vi "Open.vi"(5 "LogEnabled":bool, 7 "LogPath":path, 8 "error in (no error)":errorcluster, 9 "Instance":string, 10 "BaudRate":u32=125000, 11 "GenericCanAdapterClass in":refnum<class "GenericCanAdapterClass.lvclass">) -> (0 "error out":errorcluster, 3 "GenericCanAdapterClass out":refnum<class "GenericCanAdapterClass.lvclass">)   [LabVIEW 2011, in "GenericCanAdapterClass.lvclass"]
uses:
  GenericCanAdapterClass.lvclass
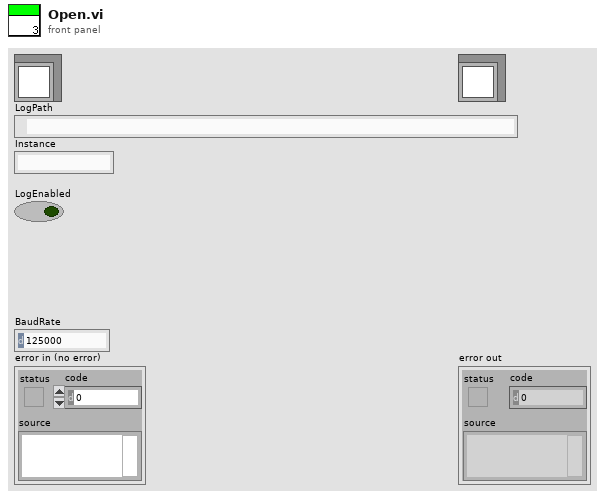
[diagram p1: front panel]
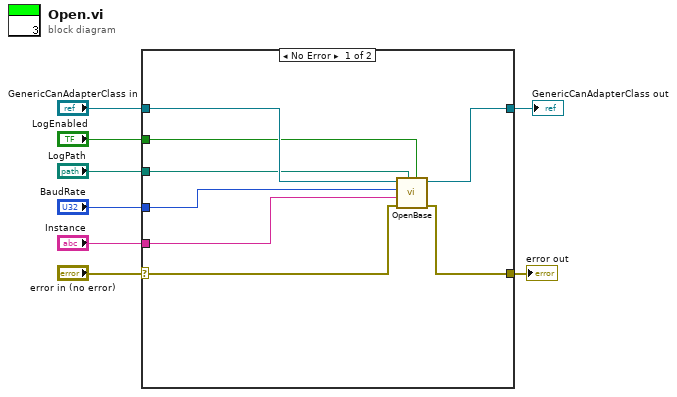
[diagram p0: block diagram]
diagram:
  n1 = case shown="No Error" "error in (no error)" {
    selector: "error in (no error)" -> [w10 w18]
    tunnel: [w9 w18] -> w7
    tunnel: [w15 w17] -> w5
    tunnel: "GenericCanAdapterClass in" -> [w16 w17]
    tunnel: "LogPath" -> [w14 _]
    tunnel: "LogEnabled" -> [w13 _]
    tunnel: "BaudRate" -> [w12 _]
    tunnel: "Instance" -> [w11 _]
    frame No Error {
      n2 = call-dynamic "OpenBase.vi"("LogEnabled"=w13, "LogPath"=w14, "error in (no error)"=w10, "Instance"=w11, "BaudRate"=w12, "GenericCanAdapterClass in"=w16) -> ("error out"=w9:errorcluster, "GenericCanAdapterClass out"=w15:refnum<class "GenericCanAdapterClass.lvclass">)  [unwired: 4 in]
    }
    frame Error {
    }
  }
  "error out" <- w7
  "GenericCanAdapterClass out" <- w5
